vi "Butterfly_Resitance w_SMU and Output Control.vi"(0 "Semiconductor Module Context":T3, 1 "script name":string="Cmax", 2 "SMU Settings":T2={"Level"=0.01, "Level Range"=0.1, "Limit"=1.0, "Limit Range"=6.0, "Sense"=0} {"Sense" items=["Local"=1008, "Remote"=1009]}, 5 "Pins":string[](array[string])=["RF"], 7 "HV_Voltages":dbl[](array[numeric]), 9 "Thresholds(max R 1st)":dbl[](array[numeric])=[100000.0, 0.5], 11 "error in (no error)":errorcluster) -> (4 "R Array":dbl[][](array[numeric]), 15 "error out":errorcluster)   [LabVIEW 2013]
uses:
  <instrlib>/niHSDIO/niHSDIO.llb/niHSDIO_ctl Trigger Script - trigID Values (Ring).ctl
  <vilib>/NI_TestStand_SemiconductorModule/NI_TestStand_Semiconductor_Module.lvlibp
  <vilib>/NI_TestStand_SemiconductorModule/NI_TestStand_Semiconductor_Module.lvlibp/PinMap/General/Publish/PublishDataDoubleFunctionalTest.vi
  <vilib>/NI_TestStand_SemiconductorModule/NI_TestStand_Semiconductor_Module.lvlibp/PinMap/DC Power/PinsToNIDCPowerSessions.vi
  <vilib>/NI_TestStand_SemiconductorModule/NI_TestStand_Semiconductor_Module.lvlibp/PinMap/General/SemiconductorModuleContext.ctl
  <instrlib>/niDCPower/nidcpower.llb/niDCPower Sense.ctl
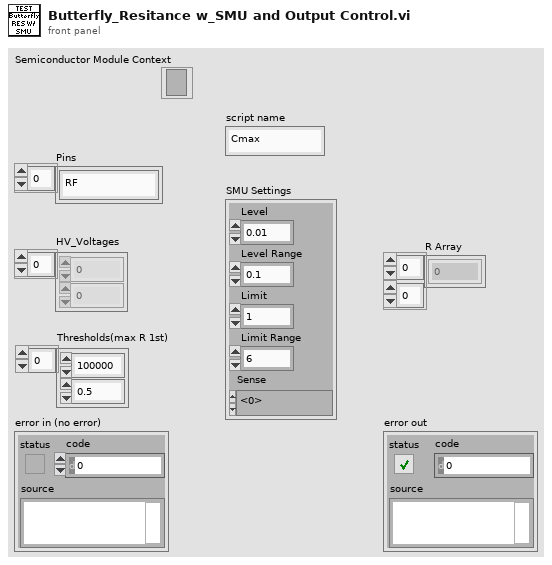
[diagram p1: front panel]
types:
  T1 = typedef "niDCPower Sense.ctl" = i32
  T2 = cluster{"Level":dbl, "Level Range":dbl, "Limit":dbl, "Limit Range":dbl, "Sense":T1}
  T3 = typedef "NI_TestStand_Semiconductor_Module.lvlibp/SemiconductorModuleContext.ctl" = refnum<k7>
  T4 = typedef "niHSDIO_ctl Trigger Script - trigID Values (Ring).ctl" = string
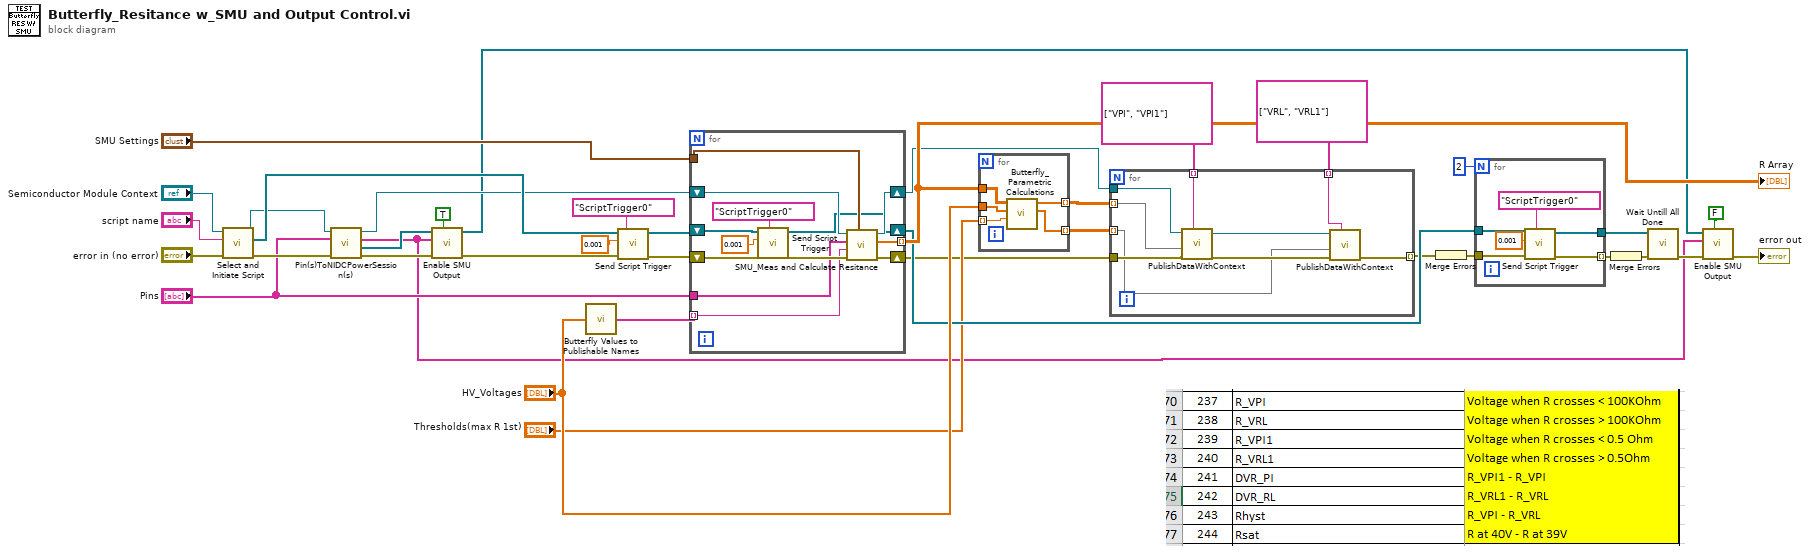
[diagram p0: block diagram]
diagram:
  n1 = call "Select and Initiate Script.vi"("error in (no error)"="error in (no error)", "script name"="script name", "Semiconductor Module Context"="Semiconductor Module Context") -> ("error out"=w12:errorcluster, "HSDIO GEN Sessions Out"=w15:refnum<k15>[], "Semiconductor Module Context Out"=w10:T3)  [unwired: 6 in]
  n2 = call-poly <vilib>:"Pin(s)ToNIDCPowerSession(s).vi"("error in (no error)"=w12, "Pins"="Pins", "Semiconductor Module Context"=w10) -> ("error out"=w13:errorcluster, "Instrument Sessions"=w7:refnum<k15>[], "Channel Lists"=w2:string[], "Semiconductor Module Context Out"=w9:T3)  [unwired: 4 in, 1 out]
  n3 = call "Enable SMU Output.vi"("output enabled"=TRUE, "error in (no error)"=w13, "Channel Lists"=w2, "Instrument Sessions In"=w7) -> ("error Out"=w11:errorcluster, "Instrument Sessions Out"=w3:refnum<k15>[])  [unwired: 6 in]
  n4 = call "Butterfly Values to Publishable Names.vi"("Butterfly Numbers"="HV_Voltages") -> ("Publishable Names"=w36:string[])
  n5 = call "Send Script Trigger.vi"("trigger id (script trigger 0)"=T4 "ScriptTrigger0", "error in (no error)"=w11, "Delay Time (s)"=0.001, "HSDIO Sessions In"=w15) -> ("error out"=w17:errorcluster, "HSDIO Sessions Out"=w16:refnum<k15>[])  [unwired: 6 in]
  n6 = for {
    shift-right: [w49] -> w27
    shift-left: w17 -> [w52]
    shift-right: [w43] -> w26
    shift-left: w9 -> [w48]
    tunnel: w36 -> [w46] mode=indexing
    tunnel: "Pins" -> [w45]
    tunnel: "SMU Settings" -> [w44]
    tunnel: [w42] -> w34 mode=indexing
    shift-right: [w40] -> w31
    shift-left: w16 -> [w41]
    n7 = call "Send Script Trigger.vi"("trigger id (script trigger 0)"=T4 "ScriptTrigger0", "error in (no error)"=w52, "Delay Time (s)"=0.001, "HSDIO Sessions In"=w41) -> ("error out"=w50:errorcluster, "HSDIO Sessions Out"=w40:refnum<k15>[])  [unwired: 6 in]
    n8 = call "SMU_Meas and Calculate Resitance.vi"("Current  Level"=w44, "error in (no error)"=w50, "Published Data Id"=w46, "Pins"=w45, "Semiconductor Module Context"=w48) -> ("error Out"=w49:errorcluster, "R Array"=w42:dbl[], "Semiconductor Module Context Out"=w43:T3)  [unwired: 4 in]
  }
  "R Array" <- w34
  n9 = for {
    tunnel: w34 -> [w57]
    tunnel: "HV_Voltages" -> [w56]
    tunnel: [w55] -> w23 mode=indexing
    tunnel: [w54] -> w22 mode=indexing
    tunnel: "Thresholds(max R 1st)" -> [w53] mode=indexing
    n10 = call "Butterfly_Parametric Calculations.vi"("Threshold"=w53, "Voltage Array"=w56, "Result Array In"=w57) -> ("VRLs"=w54:dbl[], "VPIs"=w55:dbl[])  [unwired: 7 in]
  }
  n11 = for {
    tunnel: w27 -> [w66]
    tunnel: w26 -> [w65]
    tunnel: [w63] -> w25 mode=indexing
    tunnel: w23 -> [w61] mode=indexing
    tunnel: w22 -> [w58] mode=indexing
    tunnel: string[] ["VPI", "VPI1"] -> [w60] mode=indexing
    tunnel: string[] ["VRL", "VRL1"] -> [w59] mode=indexing
    n12 = call-poly <vilib>:"PublishDataWithContext.vi"("Published Data Id"=w60, "error in (no error)"=w66, "Data In"=w61, "Semiconductor Module Context"=w65) -> ("error out"=w64:errorcluster, "Semiconductor Module Context Out"=w62:T3)  [unwired: 6 in]
    n13 = call-poly <vilib>:"PublishDataWithContext.vi"("Published Data Id"=w59, "error in (no error)"=w64, "Data In"=w58, "Semiconductor Module Context"=w62) -> ("error out"=w63:errorcluster)  [unwired: 6 in, 1 out]
  }
  n14 = Merge Errors(w25) -> (w24:errorcluster)
  n15 = for {
    N: 2 -> [_]
    tunnel: w31 -> [w72]
    tunnel: [w71] -> w30
    tunnel: [w70] -> w29 mode=indexing
    tunnel: w24 -> [w67]
    n16 = call "Send Script Trigger.vi"("trigger id (script trigger 0)"=T4 "ScriptTrigger0", "error in (no error)"=w67, "Delay Time (s)"=0.001, "HSDIO Sessions In"=w72) -> ("error out"=w70:errorcluster, "HSDIO Sessions Out"=w71:refnum<k15>[])  [unwired: 6 in]
  }
  n17 = Merge Errors(w29) -> (w32:errorcluster)
  n18 = call "Wait Untill All Done.vi"("error in (no error)"=w32, "HSDIO Sessions In"=w30) -> ("error out"=w5:errorcluster)  [unwired: 8 in, 1 out]
  n19 = call "Enable SMU Output.vi"("output enabled"=FALSE, "error in (no error)"=w5, "Channel Lists"=w2, "Instrument Sessions In"=w3) -> ("error Out"=→"error out":errorcluster)  [unwired: 6 in, 1 out]
